vi "Lock_File.vi"(3 "error in (no error)":errorcluster, 4 "Lock File":bool, 5 "path":path) -> (0 "error out":errorcluster, 2 "dup path":path)   [LabVIEW 2010]
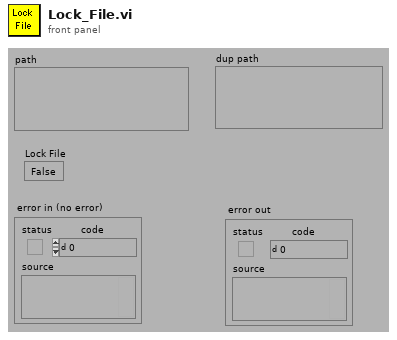
[diagram p1: front panel]
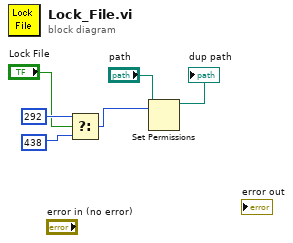
[diagram p0: block diagram]
diagram:
  n1 = Select(t=i16 292 ("new permissions"), s="Lock File", f=i16 438 ("new permissions")) -> (s? t:f=w2:i16)
  n2 = Set Permissions(7:w2, 11:"path") -> (3:→"dup path":path)  [unwired: 1 in, 3 out]
